vi "SV Multitone THD IMD SNR (Frequency) (1 Ch).vi"(0 "complex spectrum response":T12={"complex spectrum response"={"f0"=0.0, "df"=1.0, "complex spectrum"=[]}, "spectrum info"={"channel name"="", "description"="", "x-axis units"=0, "spectral info"={"spectrum type"=enum."Power [Magnitude^2]", "linear/dB"=enum."linear", "window"=0, "window size"=0, "FFT size"=0}, "engineering units"=0, "custom label"="", "dB reference [EU]"=0.0, "peak units"=enum."rms", "weighting filter"=0, "spectral density?"=FALSE, "unit label"="", "spectrum skewed?"=FALSE, "complimentary spectrum units"=enum."none"}} {"spectrum info"."x-axis units" items=["Time (s)"=0, "Frequency-CB (Hz)"=1, "Frequency-CPB (Hz)"=1248, "Frequency-Arbitrary (Hz)"=2357, "Quefrency (s)"=2, "Revolutions (rev)"=3, "Order"=4, "Speed (RPM)"=11, "Speed (rad/s)"=21, "Index"=65535]; "spectrum info"."weighting filter" items=["Linear", "A-weighting", "B-weighting", "C-weighting", "ITU-R 468-4", "Dolby", "CCITT", "C-message", "Wb", "Wc", "Wd", "We", "Wf", "Wh", "Wj", "Wk", "Wm", "AES17 20 kHz lowpass", "AES17 40 kHz lowpass", "AES17 20 kHz highpass", "AES17 40 kHz highpass"]; "spectrum info"."dB reference [EU]" format="%.2f"; "spectrum info"."engineering units" items=["custom..."=0, "V"=1, "A"=21, "C"=30, "pC"=31, "s"=32, "-"=29, "Pa"=2, "N"=20, "g"=3, "m/s^2"=4, "m/s"=5, "m"=6, "mm/s"=12, "mm"=13, "micron/s"=14, "micron"=15, "in/s^2"=7, "in/s"=8, "in"=9, "mil/s"=10, "mil"=11, "rad/s^2"=16, "rad/s"=17, "rad"=18, "deg/s^2"=26, "deg/s"=27, "deg"=28, "RPM"=22, "cycle/s^2"=23, "Hz"=24, "cycle"=25, "strain"=19]; "spectrum info"."spectral info"."window" items=["None "=0, "Hanning"=1, "Hamming"=2, "Blackman-Harris"=3, "Exact Blackman"=4, "Blackman"=5, "Flat Top"=6, "4 Term B-Harris "=7, "7 Term B-Harris"=8, "Low Sidelobe"=9, "Force - Exponential"=10, "Gaussian"=62]; "complex spectrum response"."complex spectrum" format="%.2f"; "complex spectrum response"."df" format="%.2f"; "complex spectrum response"."f0" format="%.2f"}, 1 "reference tones":T5(array[cluster]) {"phase (deg)" format="%0.3p"; "amplitude [EU pk]" format="%0.3p"; "frequency [Hz]" format="%0.3p"}, 2 "frequency range [Hz]":cluster{"start":dbl, "stop":dbl}={"start"=-1.0, "stop"=-1.0} {"stop" format="%.2f"; "start" format="%.2f"}, 3 "advanced span [Hz]":dbl=-1.0 format="%.2f", 5 "error in (no error)":errorcluster, 6 "desired units":T14={"THD"=enum."dB", "IMD"=enum."dB", "SNR"=enum."dB", "harmonic level"=enum."EU rms", "intermodulation level"=enum."EU rms", "noise level"=enum."EU rms"}, 7 "configuration":T2={"maximum harmonic"=5, "IMD proxy frequencies"=[], "noise proxy"=0} {"noise proxy" items=["Residual"=0, "L50"=50, "L75"=75, "L90"=90, "Odd bins"=13579]}) -> (12 "unit labels":T13, 13 "distortion frequencies [Hz]":T4, 14 "complex spectrum response":T12={"complex spectrum response"={"f0"=0.0, "df"=1.0, "complex spectrum"=[]}, "spectrum info"={"channel name"="", "description"="", "x-axis units"=0, "spectral info"={"spectrum type"=enum."Power [Magnitude^2]", "linear/dB"=enum."linear", "window"=0, "window size"=0, "FFT size"=0}, "engineering units"=0, "custom label"="", "dB reference [EU]"=0.0, "peak units"=enum."rms", "weighting filter"=0, "spectral density?"=FALSE, "unit label"="", "spectrum skewed?"=FALSE, "complimentary spectrum units"=enum."none"}} {"spectrum info"."x-axis units" items=["Time (s)"=0, "Frequency-CB (Hz)"=1, "Frequency-CPB (Hz)"=1248, "Frequency-Arbitrary (Hz)"=2357, "Quefrency (s)"=2, "Revolutions (rev)"=3, "Order"=4, "Speed (RPM)"=11, "Speed (rad/s)"=21, "Index"=65535]; "spectrum info"."weighting filter" items=["Linear", "A-weighting", "B-weighting", "C-weighting", "ITU-R 468-4", "Dolby", "CCITT", "C-message", "Wb", "Wc", "Wd", "We", "Wf", "Wh", "Wj", "Wk", "Wm", "AES17 20 kHz lowpass", "AES17 40 kHz lowpass", "AES17 20 kHz highpass", "AES17 40 kHz highpass"]; "spectrum info"."dB reference [EU]" format="%.2f"; "spectrum info"."engineering units" items=["custom..."=0, "V"=1, "A"=21, "C"=30, "pC"=31, "s"=32, "-"=29, "Pa"=2, "N"=20, "g"=3, "m/s^2"=4, "m/s"=5, "m"=6, "mm/s"=12, "mm"=13, "micron/s"=14, "micron"=15, "in/s^2"=7, "in/s"=8, "in"=9, "mil/s"=10, "mil"=11, "rad/s^2"=16, "rad/s"=17, "rad"=18, "deg/s^2"=26, "deg/s"=27, "deg"=28, "RPM"=22, "cycle/s^2"=23, "Hz"=24, "cycle"=25, "strain"=19]; "spectrum info"."spectral info"."window" items=["None "=0, "Hanning"=1, "Hamming"=2, "Blackman-Harris"=3, "Exact Blackman"=4, "Blackman"=5, "Flat Top"=6, "4 Term B-Harris "=7, "7 Term B-Harris"=8, "Low Sidelobe"=9, "Force - Exponential"=10, "Gaussian"=62]; "complex spectrum response"."complex spectrum" format="%.2f"; "complex spectrum response"."df" format="%.2f"; "complex spectrum response"."f0" format="%.2f"}, 15 "THD":dbl format="%.2f", 16 "IMD":dbl format="%.2f", 17 "SNR":dbl format="%.2f", 18 "levels":T3 {"noise" format="%.2f"; "intermodulation" format="%.2f"; "harmonic" format="%.2f"}, 19 "error out":errorcluster)   [LabVIEW 2017, in "SoundVib_Multitone.lvlib"]
doc: "Performs total harmonic distortion (THD), intermodulation distortion (IMD), and signal-to-noise ratio (SNR) measurements, including measuring the fundamental tones, harmonic components, intermodulation components, and residual noise. Wire data to the <B>scaled signal [EU]</B> input to determine the polymorphic instance to use or manually select the instance."
uses:
  <vilib>/addons/Sound and Vibration/svt_Multitone Distortion/SoundVib_Multitone.lvlib
  <vilib>/addons/_NISVFA/_Shared subVIs/Controls/svc_Spectrum Info.ctl
  <vilib>/addons/_NISVFA/_Shared subVIs/Controls/svc_X-Axis Units.ctl
  <vilib>/addons/_NISVFA/_Shared subVIs/Controls/svc_Spectrum Type.ctl
  <vilib>/addons/_NISVFA/_Shared subVIs/Controls/svc_Engineering Units Text Ring.ctl
  <vilib>/addons/_NISVFA/_Shared subVIs/Controls/svc_Weighting Filter Text Ring.ctl
  <vilib>/addons/_NISVFA/_Shared subVIs/Controls/svc_Complimentary Spectrum Units.ctl
  <vilib>/addons/_NISVFA/_Shared subVIs/Controls/svc_Noise Proxy.ctl
  <vilib>/addons/_NISVFA/_Spectrum Processing/SVFA Power in Band (1 Ch).vi
  <vilib>/addons/_NISVFA/_Spectrum Processing/SVFA Get Spectrum Subset (1 Ch).vi
  <vilib>/addons/_NISVFA/_Shared subVIs/Common/svc_Spectrum Units.vi
  <vilib>/addons/_NISVFA/_Spectrum Processing/SVFA Unit Conversion (1 Ch).vi
  <vilib>/addons/_NISVFA/_Spectrum Processing/subVIs/svfa_Conversion Utility (spectrum info).vi
  <vilib>/addons/_NISVFA/_Spectrum Processing/subVIs/svfa_Peak to RMS to Peak2Peak.vi
  <vilib>/addons/_NISVFA/_Spectrum Processing/subVIs/svfa_Mag to Mag2.vi
  <vilib>/addons/_NISVFA/_Spectrum Processing/subVIs/svfa_Linear to dB.vi
  <vilib>/addons/_NISVFA/_Spectrum Processing/subVIs/svfa_dBrefA to dBrefB.vi
  <vilib>/addons/_NISVFA/_Spectrum Processing/subVIs/svfa_Spectrum to Spectral Density.vi
  <vilib>/addons/_NISVFA/_Shared subVIs/Common/svc_Get Weighting Enum and Labels.vi
  <vilib>/addons/_NISVFA/_Shared subVIs/Common/svc_Unit Label Lexical Class.vi
  <vilib>/addons/_NISVFA/_Shared subVIs/Common/svc_Engineering Units to Unit Label.vi
  <vilib>/addons/_NISVFA/_Shared subVIs/Common/svc_Format Value (DBL).vi
  <vilib>/addons/_NISVFA/_Shared subVIs/Common/svc_Window Parameters.vi
  <vilib>/addons/_NISVFA/_Spectrum Processing/subVIs/svfa_Spectrum Info Window to windowTd Type Def.vi
  <vilib>/addons/_NISVFA/_Shared subVIs/Common/svc_Build Unit Label for Frequency Range.vi
  <vilib>/addons/_NISVFA/_Shared subVIs/Common/svc_Convert Frequency to Frequency String.vi
  <vilib>/addons/_NISVFA/_Shared subVIs/Common/svc_Check Frequency Range in Spectrum.vi
  <vilib>/addons/_NISVFA/_Spectrum Processing/SVFA Unit Conversion (Complex) (1 Ch).vi
  <vilib>/addons/_NISVFA/_Spectrum Processing/SVFA Get Spectrum Subset (Complex) (1 Ch).vi
  <vilib>/addons/Sound and Vibration/svt_Distortion/SoundVib_Distortion.lvlib
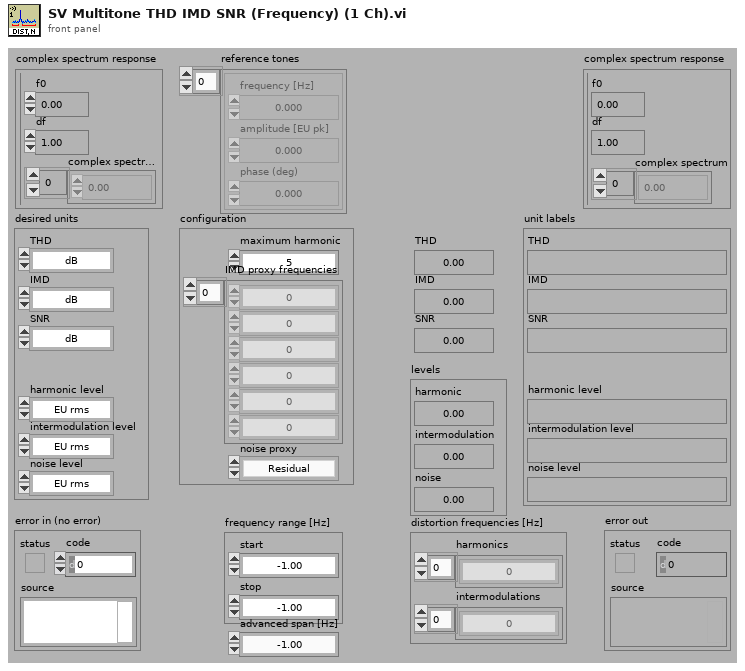
[diagram p1: front panel]
types:
  T1 = typedef "svc_Noise Proxy.ctl" = u16
  T2 = cluster{"maximum harmonic":i32, "IMD proxy frequencies":dbl[], "noise proxy":T1}
  T3 = cluster{"harmonic":dbl, "intermodulation":dbl, "noise":dbl}
  T4 = cluster{"harmonics":dbl[], "intermodulations":dbl[]}
  T5 = cluster{"frequency [Hz]":dbl, "amplitude [EU pk]":dbl, "phase (deg)":dbl}[]
  T6 = typedef "svc_Spectrum Info.ctl" = cluster{"channel name":string, "description":string, "x-axis units":T7, "spectral info":cluster{"spectrum type":T8, "linear/dB":enum16{"linear", "dB"}, "window":u16, "window size":i32, "FFT size":i32}, "engineering units":T9, "custom label":string, "dB reference [EU]":dbl, "peak units":enum16{"rms", "peak", "peak-peak"}, "weighting filter":T10, "spectral density?":bool, "unit label":string, "spectrum skewed?":bool, "complimentary spectrum units":T11}
  T7 = typedef "svc_X-Axis Units.ctl" = u16
  T8 = typedef "svc_Spectrum Type.ctl" = enum16{"FFT Spectrum [complex]", "Amplitude [Magnitude]", "Power [Magnitude^2]", "Cross Spectrum [complex]", "Frequency Response [Complex]"}
  T9 = typedef "svc_Engineering Units Text Ring.ctl" = u16
  T10 = typedef "svc_Weighting Filter Text Ring.ctl" = u16
  T11 = typedef "svc_Complimentary Spectrum Units.ctl" = enum16{"none", "radians", "degrees", "cycles", "imaginary"}
  T12 = cluster{"complex spectrum response":cluster{"f0":dbl, "df":dbl, "complex spectrum":cdb[]}, "spectrum info":T6}
  T13 = cluster{"THD":string, "IMD":string, "SNR":string, "harmonic level":string, "intermodulation level":string, "noise level":string}
  T14 = cluster{"THD":enum16{"dB", "linear ratio", "%"}, "IMD":enum16{"dB", "linear ratio", "%"}, "SNR":enum16{"dB", "linear ratio", "%"}, "harmonic level":enum16{"EU^2 rms", "EU rms", "dB", "dBc", "dBV", "dBu", "dBm"}, "intermodulation level":enum16{"EU^2 rms", "EU rms", "dB", "dBc", "dBV", "dBu", "dBm"}, "noise level":enum16{"EU^2 rms", "EU rms", "dB", "dBc", "dBV", "dBu", "dBm"}}
  T15 = enum32{"none", "input signal", "detected signal", "residual signal"}
  T16 = cluster{"linear/dB":enum16{"no change", "linear", "dB"}, "dB reference (0: no change)":dbl, "power/magnitude":enum16{"no change", "power", "magnitude"}, "view":enum16{"no change", "rms", "peak", "peak-peak"}}
  T17 = cluster{"frequency [Hz]":dbl, "amplitude [EU pk]":dbl, "phase [deg]":dbl}[]
  T18 = cluster{"complex spectrum subset":cluster{"x0":dbl, "dx":dbl, "complex array":cdb[]}, "spectrum info":T6}
  T19 = cluster{"frequency [Hz]":dbl, "amplitude [EU pk]":dbl, "phase [deg]":dbl}
  T20 = enum16{"EU^2 rms", "EU rms", "dB", "dBc", "dBV", "dBu", "dBm"}
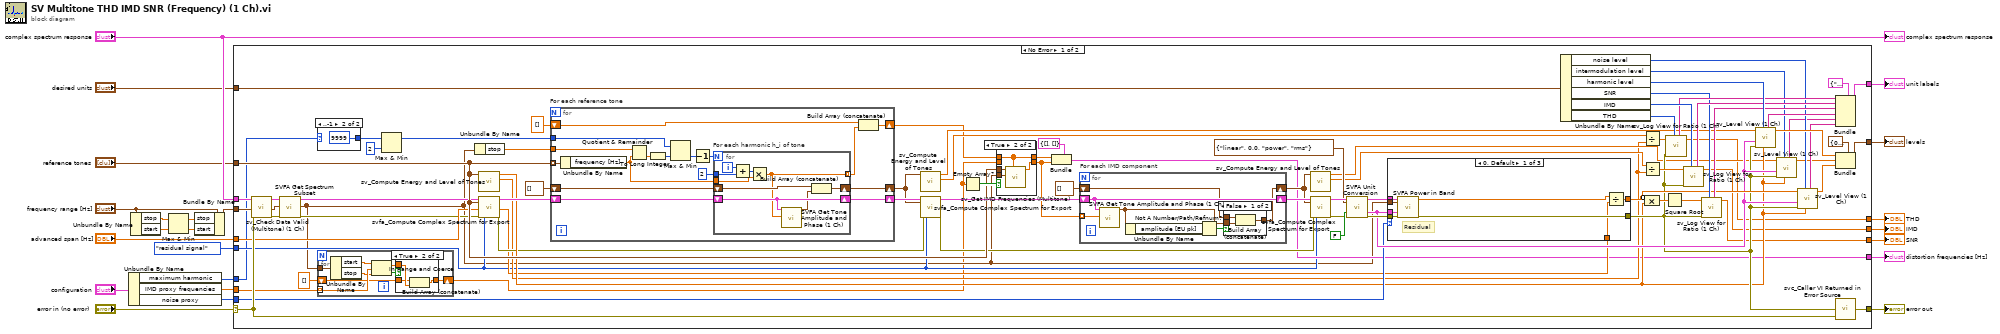
[diagram p0: block diagram]
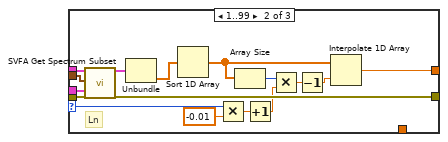
[diagram p4: hidden frame]
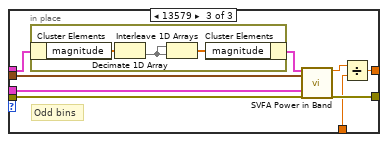
[diagram p5: hidden frame]
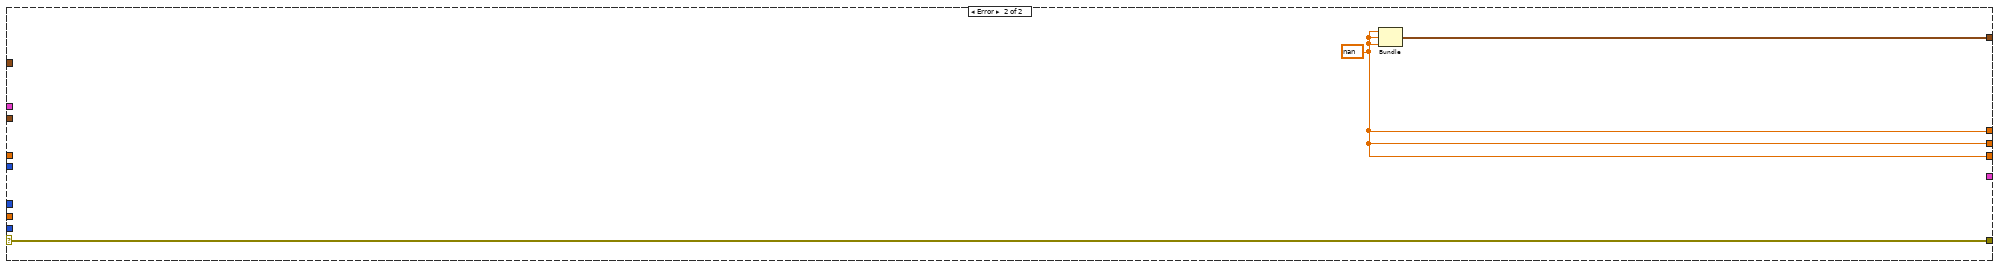
[diagram p8: hidden frame]
diagram:
  n1 = Unbundle By Name("configuration") -> ("maximum harmonic"=w1:i32, "IMD proxy frequencies"=w3:dbl[], "noise proxy"=w4:T1)
  n2 = Unbundle By Name("frequency range [Hz]") -> ("stop"=w17:dbl, "start"=w14:dbl)
  n3 = Max & Min(x=w17, y=w14) -> (max(x,y)=w16:dbl, min(x,y)=w15:dbl)
  n4 = Bundle By Name(cluster="frequency range [Hz]", "stop"=w16, "start"=w15) -> (w18:cluster{"start":dbl, "stop":dbl})
  n5 = case shown="No Error" "error in (no error)" {
    selector: "error in (no error)" -> [w102 w200]
    tunnel: "complex spectrum response" -> [w103 _]
    tunnel: [w105 w200] -> w22
    tunnel: "desired units" -> [w104 _]
    tunnel: "reference tones" -> [w57 _]
    tunnel: w18 -> [w100 _]
    tunnel: [w79 _] -> w13
    tunnel: w3 -> [w30 _]
    tunnel: [w35 _] -> w12
    tunnel: [w68 w199] -> w11
    tunnel: T15."residual signal" ("export signals") -> [w33 _]
    tunnel: w4 -> [w53 _]
    tunnel: [w45 w198] -> w9
    tunnel: [w44 w198] -> w8
    tunnel: [w43 w198] -> w7
    tunnel: "advanced span [Hz]" -> [w42 _]
    tunnel: w1 -> [w26 _]
    frame No Error {
      n6 = call <vilib>:"sv_Check Data Valid (Multitone) (1 Ch).vi"("complex spectrum"=w103, "frequency range in [Hz]"=w100, "error in (no error)"=w102) -> ("complex spectrum"=w40:T12, "frequency range out [Hz]"=w38:cluster{"start":dbl, "stop":dbl}, "error out"=w37:errorcluster)  [unwired: 14 in]
      n7 = call-poly <vilib>:"SVFA Get Spectrum Subset.vi"("complex spectrum"=w40, "range"=w38, "error in (no error)"=w37) -> ("complex spectrum subset"=w39:T18, "actual range"=w32:cluster{"start":dbl, "stop":dbl}, "error out"=w36:errorcluster)  [unwired: 13 in, 1 out]
      n8 = case shown="..-1" w26 {
        selector: w26 -> [w106 _]
        tunnel: [w106 9999 ("maximum harmonic")] -> w28
        frame Default {
        }
        frame ..-1 {
        }
      }
      n9 = for {
        tunnel: w32 -> [w115]
        tunnel: w30 -> [w113] mode=indexing
        shift-right: [w109] -> w29
        shift-left: dbl[] [] -> [w108]
        n10 = Unbundle By Name(w115) -> ("start"=w114:dbl, "stop"=w112:dbl)
        n11 = In Range and Coerce(upper limit=w114, x=w113, lower limit=w112) -> (coerced(x)=w110:dbl, In Range?=w111:bool)
        n12 = case shown="True" w111 {
          tunnel: w110 -> [_ w119]
          tunnel: [w116 w118] -> w109
          tunnel: w108 -> [w116 w117]
          frame False {
          }
          frame True {
            n13 = Build Array (concatenate)(w117, w119) -> (w118:dbl[])
          }
        }
      }
      n14 = Max & Min(x=w28, y=2) -> (max(x,y)=w25:i32)  [unwired: 1 out]
      n15 = Unbundle By Name(w32) -> ("stop"=w99:dbl)
      n16 = call <vilib>:"sv_Compute Energy and Level of Tones.vi"("reference tones"=w57) -> ("level [EU rms]"=w46:dbl, "energy level [EU^2 rms]"=w51:dbl)  [unwired: 9 in]
      n17 = call <vilib>:"svfa_Compute Complex Spectrum for Export.vi"("complex spectrum in"=w39, "tones"=w57, "advanced span [Hz]"=w42, "error in"=w36, "export signals"=w33) -> ("complex spectrum out"=w101:T12, "residual bandwidth ratio"=w41:dbl, "error out"=w49:errorcluster)  [unwired: 12 in]
      n18 = for "For each reference tone" {
        tunnel: w57 -> [w188] mode=indexing
        shift-right: [w185] -> w97
        shift-left: w101 -> [w187]
        tunnel: w99 -> [w186]
        shift-right: [w183] -> w56
        shift-left: T17 [] -> [w184]
        shift-right: [w179] -> w52
        shift-left: dbl[] [] -> [w182]
        tunnel: w25 -> [w175]
        n19 = Unbundle By Name(w188) -> ("frequency [Hz]"=w181:dbl)
        n20 = Quotient & Remainder(x=w186, y=w181) -> (floor(x/y)=w178:dbl)  [unwired: 1 out]
        n21 = To Long Integer(number=w178) -> (32bit integer=w174:i32)
        n22 = Max & Min(x=w175, y=w174) -> (min(x,y)=w176:i32)  [unwired: 1 out]
        n23 = Decrement(x=w176) -> (x-1=w173:i32)
        n24 = for "For each harmonic h_i of tone" {
          N: w173 -> [_]
          tunnel: 2 ("x") -> [w196]
          tunnel: w181 -> [w195]
          shift-right: [w194] -> w185
          shift-left: w187 -> [w194]
          shift-right: [w191] -> w183
          shift-left: w184 -> [w193]
          tunnel: [w190] -> w180 mode=indexing
          i -> [w197]
          n25 = Add(x=w197, y=w196) -> (x+y=w189:i32)
          n26 = Multiply(x=w189, y=w195) -> (x*y=w190:dbl)
          n27 = call <vilib>:"SVFA Get Tone Amplitude and Phase (1 Ch).vi"("complex spectrum"=w194, "tone frequency [Hz]"=w190) -> ("identified tone"=w192:T19)  [unwired: 16 in, 1 out]
          n28 = Build Array (concatenate)(w193, w192) -> (w191:T17)
        }
        n29 = Build Array (concatenate)(w182, w180) -> (w179:dbl[])
      }
      n30 = call <vilib>:"sv_Compute Energy and Level of Tones.vi"("reference tones"=w56) -> ("level [EU rms]"=w67:dbl, "energy level [EU^2 rms]"=w59:dbl)  [unwired: 9 in]
      n31 = call <vilib>:"svfa_Compute Complex Spectrum for Export.vi"("complex spectrum in"=w97, "tones"=w56, "error in"=w49, "export signals"=w33) -> ("complex spectrum out"=w95:T12, "error out"=w50:errorcluster)  [unwired: 13 in, 1 out]
      n32 = Empty Array?(array=w29) -> (empty?=w78:bool)
      n33 = case shown="True" w78 {
        tunnel: w52 -> [w156 w158]
        tunnel: [w157 w161] -> w73
        tunnel: w57 -> [_ w160]
        tunnel: w32 -> [_ w159]
        tunnel: w29 -> [w157 _]
        tunnel: [w156 w158] -> w34
        frame False {
        }
        frame True {
          n34 = call <vilib>:"sv_Get IMD Frequencies (Multitone).vi"("harmonic frequencies [Hz]"=w158, "frequency range [Hz]"=w159, "reference tones"=w160) -> ("intermodulation frequencies"=w161:dbl[])  [unwired: 8 in]
        }
      }
      n35 = Bundle(cluster=T4 {"harmonics"=[], "intermodulations"=[]} ("distortion frequencies [Hz]"), "harmonics"=w34, "intermodulations"=w73) -> (w35:T4)
      n36 = for "For each IMD component" {
        shift-right: [w168] -> w93
        shift-left: w95 -> [w168]
        shift-right: [w166] -> w55
        shift-left: T17 [] -> [w167]
        tunnel: w73 -> [w165] mode=indexing
        n37 = call <vilib>:"SVFA Get Tone Amplitude and Phase (1 Ch).vi"("complex spectrum"=w168, "tone frequency [Hz]"=w165) -> ("identified tone"=w162:T19)  [unwired: 16 in, 1 out]
        n38 = Unbundle By Name(w162) -> ("amplitude [EU pk]"=w164:dbl)
        n39 = Not A Number/Path/Refnum?(number/path/refnum=w164) -> (NaN/Path/Refnum?=w163:bool)
        n40 = case shown="False" w163 {
          tunnel: w167 -> [w171 w172]
          tunnel: [w170 w172] -> w166
          tunnel: w162 -> [w169 _]
          frame False {
            n41 = Build Array (concatenate)(w171, w169) -> (w170:T17)
          }
          frame True {
          }
        }
      }
      n42 = call <vilib>:"sv_Compute Energy and Level of Tones.vi"("reference tones"=w55) -> ("level [EU rms]"=w47:dbl, "energy level [EU^2 rms]"=w48:dbl)  [unwired: 9 in]
      n43 = call <vilib>:"svfa_Compute Complex Spectrum for Export.vi"("complex spectrum in"=w93, "tones"=w55, "error in"=w50, "export signals"=w33) -> ("complex spectrum out"=w90:T12, "error out"=w87:errorcluster)  [unwired: 13 in, 1 out]
      n44 = call-poly <vilib>:"SVFA Unit Conversion.vi"("complex spectrum"=w90, "desired scaling"=T16 {"linear/dB"=enum."linear", "dB reference (0: no change)"=0.0, "power/magnitude"=enum."power", "view"=enum."rms"}, "convert to degree (T)"=FALSE, "error in (no error)"=w87) -> ("converted spectrum"=w92:cluster{"x0":dbl, "dx":dbl, "magnitude":dbl[]}, "spectrum info out"=w58:T6, "error out"=w91:errorcluster)  [unwired: 10 in, 3 out]
      n45 = case shown="0, Default" w53 {
        selector: w53 -> [_ w129 _]
        tunnel: w92 -> [w127 w143 w152]
        tunnel: w91 -> [w126 w142 w150]
        tunnel: w32 -> [w125 w141 w149]
        tunnel: [w120 w128 w144] -> w60
        tunnel: w58 -> [w124 w140 w151]
        tunnel: [w123 w139 w147] -> w54
        tunnel: w41 -> [w122 _ w145]
        frame 0, Default {
          # "Residual"
          n46 = call-poly <vilib>:"SVFA Power in Band.vi"("spectrum"=w127, "range"=w125, "spectrum info"=w124, "error in (no error)"=w126) -> ("power in band"=w121:dbl, "error out"=w123:errorcluster)  [unwired: 13 in, 1 out]
          n47 = Divide(x=w121, y=w122) -> (x/y=w120:dbl)
        }
        frame 1..99 {
          # "Ln"
          n48 = call-poly <vilib>:"SVFA Get Spectrum Subset.vi"("spectrum"=w143, "range"=w141, "spectrum info"=w140, "error in (no error)"=w142) -> ("spectrum subset"=w138:cluster{"x0":dbl, "dx":dbl, "magnitude":dbl[]}, "error out"=w139:errorcluster)  [unwired: 10 in, 4 out]
          n49 = Unbundle(w138) -> ("magnitude"=w130:dbl[])  [unwired: 2 out]
          n50 = Sort 1D Array(array=w130) -> (sorted array=w137:dbl[])
          n51 = Multiply(x=w129, y=-0.01) -> (x*y=w132:dbl)
          n52 = Array Size(array=w137) -> (size(s)=w135:i32)
          n53 = Increment(x=w132) -> (x+1=w133:dbl)
          n54 = Multiply(x=w135, y=w133) -> (x*y=w134:dbl)
          n55 = Decrement(x=w134) -> (x-1=w136:dbl)
          n56 = Interpolate 1D Array(1:w136, 2:w137) -> (0:w128:dbl)
        }
        frame 13579 {
          # "Odd bins"
          n57 = in-place {
            n58 = in-place-cluster #1(w152) -> ("magnitude"=w155:dbl[])
            n59 = Decimate 1D Array(w155) -> (w153:dbl[])  [unwired: 1 out]
            n60 = Interleave 1D Arrays(w153, w153) -> (w154:dbl[])
            n61 = in-place-cluster #1("magnitude"=w154) -> (w148:cluster{"x0":dbl, "dx":dbl, "magnitude":dbl[]})
          }
          n62 = call-poly <vilib>:"SVFA Power in Band.vi"("spectrum"=w148, "range"=w149, "spectrum info"=w151, "error in (no error)"=w150) -> ("power in band"=w146:dbl, "error out"=w147:errorcluster)  [unwired: 13 in, 1 out]
          n63 = Divide(x=w146, y=w145) -> (x/y=w144:dbl)
        }
      }
      n64 = Unbundle By Name(w104) -> ("noise level"=w65:T20, "intermodulation level"=w64:T20, "harmonic level"=w83:T20, "SNR"=w76:enum16{"dB", "linear ratio", "%"}, "IMD"=w86:enum16{"dB", "linear ratio", "%"}, "THD"=w84:enum16{"dB", "linear ratio", "%"})
      n65 = Divide(x=w67, y=w46) -> (x/y=w82:dbl)
      n66 = Divide(x=w47, y=w46) -> (x/y=w85:dbl)
      n67 = Compound Arithmetic op=MULTIPLY(invert w60, w51) -> (w77:dbl)
      n68 = Square Root(x=w77) -> (sqrt(x)=w24:dbl)
      n69 = call <vilib>:"sv_Log View for Ratio (1 Ch).vi"("ratio units"=w84, "error in (no error)"=w54, "linear ratio"=w82) -> ("converted ratio"=w45:dbl, "unit label"=w81:string)  [unwired: 6 in, 1 out]
      n70 = call <vilib>:"sv_Log View for Ratio (1 Ch).vi"("ratio units"=w86, "error in (no error)"=w54, "linear ratio"=w85) -> ("converted ratio"=w44:dbl, "unit label"=w80:string)  [unwired: 6 in, 1 out]
      n71 = call <vilib>:"sv_Log View for Ratio (1 Ch).vi"("ratio units"=w76, "error in (no error)"=w54, "linear ratio"=w24) -> ("converted ratio"=w43:dbl, "unit label"=w74:string)  [unwired: 6 in, 1 out]
      n72 = call <vilib>:"sv_Level View (1 Ch).vi"("carrier level [EU^2 rms]"=w51, "desired units"=w83, "error in (no error)"=w54, "spectrum info"=w58, "level [EU^2 rms]"=w59) -> ("converted level"=w66:dbl, "unit label"=w75:string)  [unwired: 4 in, 1 out]
      n73 = call <vilib>:"sv_Level View (1 Ch).vi"("carrier level [EU^2 rms]"=w51, "desired units"=w64, "error in (no error)"=w54, "spectrum info"=w58, "level [EU^2 rms]"=w48) -> ("converted level"=w61:dbl, "unit label"=w62:string)  [unwired: 4 in, 1 out]
      n74 = call <vilib>:"sv_Level View (1 Ch).vi"("carrier level [EU^2 rms]"=w51, "desired units"=w65, "error in (no error)"=w54, "spectrum info"=w58, "level [EU^2 rms]"=w60) -> ("converted level"=w70:dbl, "unit label"=w63:string)  [unwired: 4 in, 1 out]
      n75 = Bundle(cluster=T13 {"THD"="", "IMD"="", "SNR"="", "harmonic level"="", "intermodulation level"="", "noise level"=""} ("unit labels"), "THD"=w81, "IMD"=w80, "SNR"=w74, "harmonic level"=w75, "intermodulation level"=w62, "noise level"=w63) -> (w79:T13)
      n76 = Bundle(cluster=T3 {"harmonic"=0.0, "intermodulation"=0.0, "noise"=0.0} ("levels"), "harmonic"=w66, "intermodulation"=w61, "noise"=w70) -> (w68:T3)
      n77 = call <vilib>:"svc_Caller VI Returned in Error Source.vi"("warning input to caller"=w102, "error in (no error)"=w54) -> ("error out"=w105:errorcluster)  [unwired: 3 in]
    }
    frame Error {
      w198 = nan ("SINAD")
      n78 = Bundle("SINAD"=w198, "SINAD"=w198, "SINAD"=w198) -> (w199:cluster{"SINAD":dbl, "SINAD":dbl, "SINAD":dbl})  [unwired: 1 in]
    }
  }
  "error out" <- w22
  "unit labels" <- w13
  "distortion frequencies [Hz]" <- w12
  "levels" <- w11
  "THD" <- w9
  "IMD" <- w8
  "SNR" <- w7
  "complex spectrum response" <- "complex spectrum response"
